vi "Odour_bottle_volatilities.vi"(11 "Odour bottles":T1(array[cluster])) -> (3 "Array":dbl[](array[numeric]))   [LabVIEW 2016]
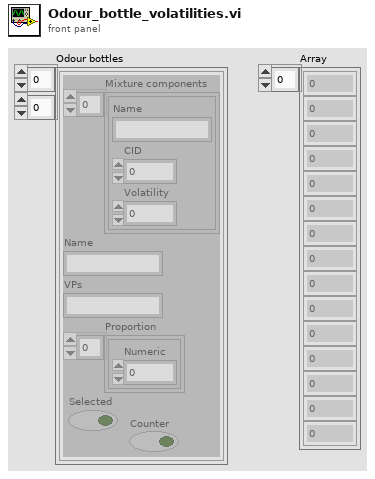
[diagram p1: front panel]
types:
  T1 = cluster{"Mixture components":cluster{"Name":string, "CID":i32, "Volatility":dbl}[], "Name":string, "VPs":string, "Proportion":cluster{"Numeric":dbl}[], "Selected":bool, "Counter":bool}[][]
  T2 = cluster{"Mixture components":cluster{"Name":string, "CID":i32, "Volatility":dbl}[], "Name":string, "VPs":string, "Proportion":cluster{"Numeric":dbl}[], "Selected":bool, "Counter":bool}[]
  T3 = cluster{"Mixture components":cluster{"Name":string, "CID":i32, "Volatility":dbl}[], "Name":string, "VPs":string, "Proportion":cluster{"Numeric":dbl}[], "Selected":bool, "Counter":bool}
  T4 = cluster{"Name":string, "CID":i32, "Volatility":dbl}[]
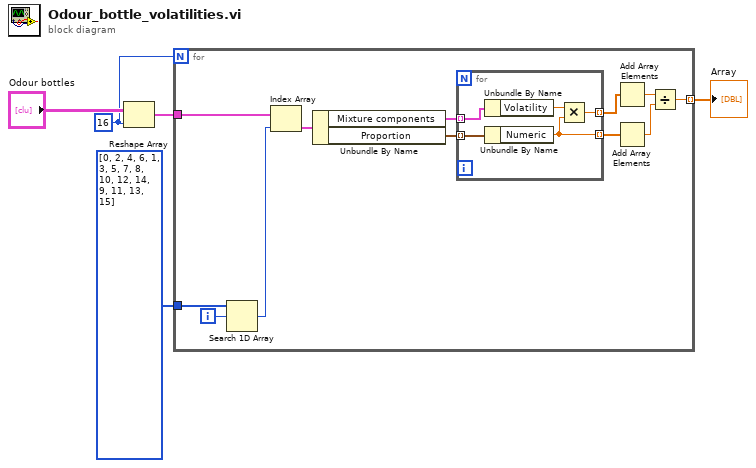
[diagram p0: block diagram]
diagram:
  w1 = 16 ("dimension size")
  n1 = Reshape Array("Odour bottles", w1) -> (w3:T2)
  n2 = for {
    N: w1 -> [_]
    tunnel: w3 -> [w10]
    tunnel: [w11] -> w5 mode=indexing
    tunnel: i32[] [0, 2, 4, 6, 1, 3, 5, 7, 8, 10, 12, 14, 9, 11, 13, 15] -> [w9]
    i -> [w8]
    n3 = Search 1D Array(1D array=w9, element=w8) -> (index of element=w7:i32)  [unwired: 1 in]
    n4 = Index Array(array=w10, index=w7) -> (element=w6:T3)
    n5 = Unbundle By Name(w6) -> ("Mixture components"=w17:T4, "Proportion"=w16:cluster{"Numeric":dbl}[])
    n6 = for {
      tunnel: w17 -> [w22] mode=indexing
      tunnel: [w20] -> w15 mode=indexing
      tunnel: w16 -> [w21] mode=indexing
      tunnel: [w18] -> w13 mode=indexing
      n7 = Unbundle By Name(w22) -> ("Volatility"=w19:dbl)
      n8 = Unbundle By Name(w21) -> ("Numeric"=w18:dbl)
      n9 = Multiply(x=w19, y=w18) -> (x*y=w20:dbl)
    }
    n10 = Add Array Elements(numeric array=w15) -> (sum=w14:dbl)
    n11 = Add Array Elements(numeric array=w13) -> (sum=w12:dbl)
    n12 = Divide(x=w14, y=w12) -> (x/y=w11:dbl)
  }
  "Array" <- w5
